vi "Data step til GUI step.vi"(7 "data step cluster":T5) -> (6 "Enabled":bool, 8 "GUI step clluster":T1)   [LabVIEW 2011]
uses:
  Sequence steps config..ctl
  Single criteria cluster.ctl
  Criteria types.ctl
  Boolean operation.ctl
  Sequence step GUI.ctl
  X-cont Action select/Action select.xctl
  X-cont criteria/Criteria control.xctl
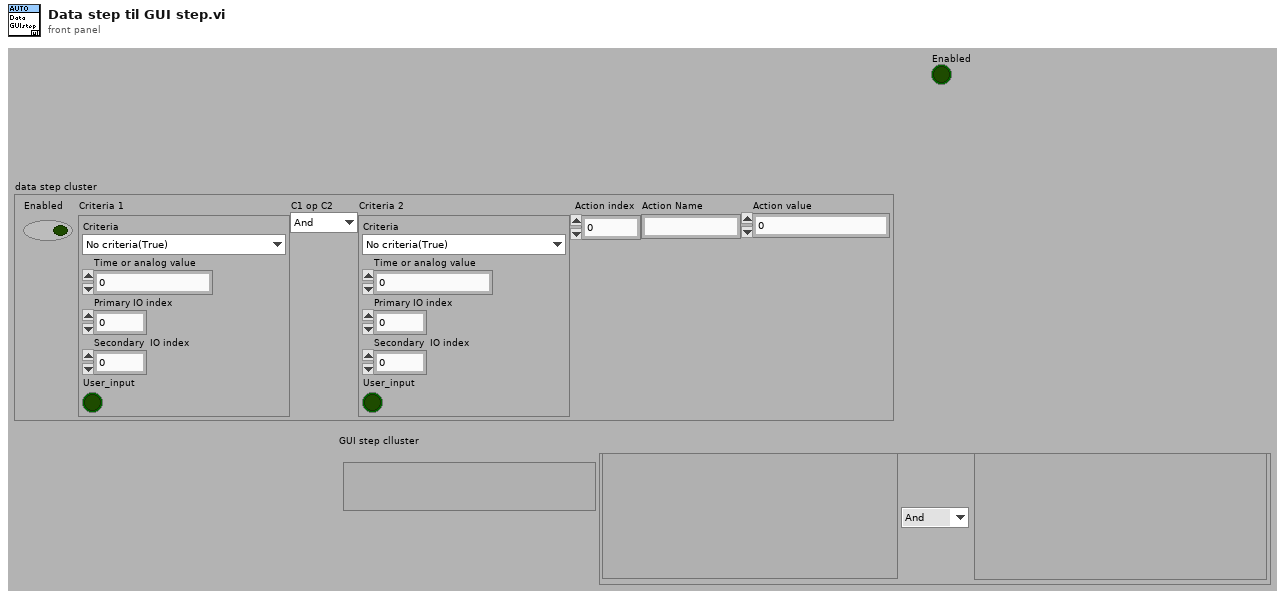
[diagram p1: front panel]
types:
  T1 = typedef "Sequence step GUI.ctl" = cluster{"Action select":cluster{"Action index":i32, "Data":dbl}, "Criteria 1":cluster{"Criteria":T2}, "C1 op C2":T4, "Criteria 2":cluster{"Criteria":T2}}
  T2 = typedef "Single criteria cluster.ctl" = cluster{"Criteria":T3, "Time or analog value":dbl, "Primary IO index":i32, "Secondary  IO index":i32, "User_input":bool}
  T3 = typedef "Criteria types.ctl" = enum16{"No criteria(True)", "Time(s)", "Analog IO over", "Analog IO over or equal", "Analog IO under", "Analog IO under or equal", "Analog IO 1 minus Analog IO 2 over", "Digital IO True", "Digital IO False", "Operator approval"}
  T4 = typedef "Boolean operation.ctl" = enum16{"And", "Or", "Xor", "Nand", "Nor", "Nxor", "Implies"}
  T5 = typedef "Sequence steps config..ctl" = cluster{"Enabled":bool, "Criteria 1":T2, "C1 op C2":T4, "Criteria 2":T2, "Action index":i32, "Action Name":string, "Action value":dbl}
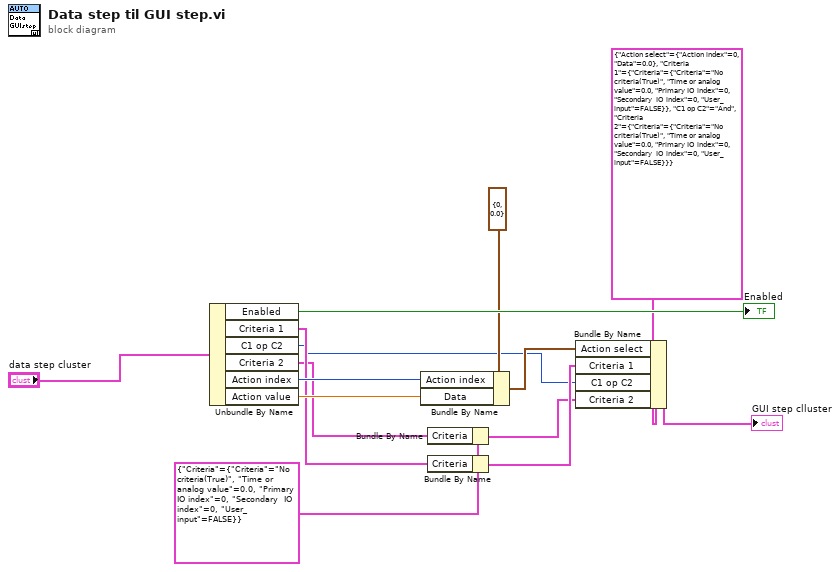
[diagram p0: block diagram]
diagram:
  w4 = cluster{"Criteria":T2} {"Criteria"={"Criteria"=enum."No criteria(True)", "Time or analog value"=0.0, "Primary IO index"=0, "Secondary  IO index"=0, "User_input"=FALSE}} ("Criteria 1")
  n1 = Unbundle By Name("data step cluster") -> ("Enabled"=→"Enabled":bool, "Criteria 1"=w6:T2, "C1 op C2"=w1:T4, "Criteria 2"=w3:T2, "Action index"=w8:i32, "Action value"=w7:dbl)
  n2 = Bundle By Name(cluster=cluster{"Action index":i32, "Data":dbl} {"Action index"=0, "Data"=0.0} ("Action select"), "Action index"=w8, "Data"=w7) -> (w9:cluster{"Action index":i32, "Data":dbl})
  n3 = Bundle By Name(cluster=w4, "Criteria"=w3) -> (w2:cluster{"Criteria":T2})
  n4 = Bundle By Name(cluster=w4, "Criteria"=w6) -> (w5:cluster{"Criteria":T2})
  n5 = Bundle By Name(cluster=T1 {"Action select"={"Action index"=0, "Data"=0.0}, "Criteria 1"={"Criteria"={"Criteria"=enum."No criteria(True)", "Time or analog value"=0.0, "Primary IO index"=0, "Secondary  IO index"=0, "User_input"=FALSE}}, "C1 op C2"=enum."And", "Criteria 2"={"Criteria"={"Criteria"=enum."No criteria(True)", "Time or analog value"=0.0, "Primary IO index"=0, "Secondary  IO index"=0, "User_input"=FALSE}}} ("GUI step clluster"), "Action select"=w9, "Criteria 1"=w5, "C1 op C2"=w1, "Criteria 2"=w2) -> (→"GUI step clluster":T1)
